vi "Logger Remove Last Log Element.vi"(8 "error in (no error)":errorcluster, 11 "LoggerRef In":T1) -> (0 "error out":errorcluster, 2 "Element Removed":string, 3 "LoggerRef Out":T1)   [LabVIEW 2014]
uses:
  LoggerRef.ctl
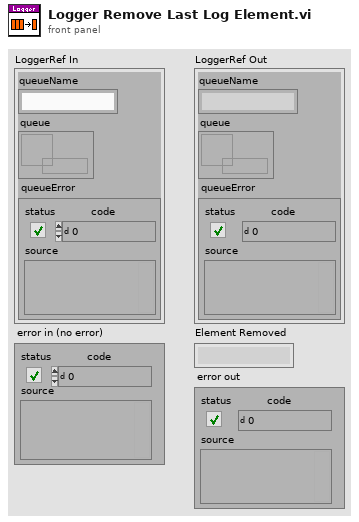
[diagram p1: front panel]
types:
  T1 = typedef "LoggerRef.ctl" = cluster{"queueName":string, "queue":refnum<queue>, "queueError":errorcluster}
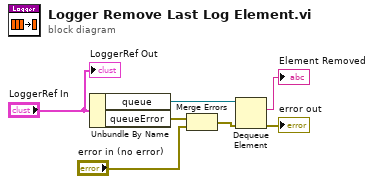
[diagram p0: block diagram]
diagram:
  n1 = Unbundle By Name("LoggerRef In") -> ("queue"=w4:refnum<queue>, "queueError"=w7:errorcluster)
  n2 = Merge Errors(w7, "error in (no error)") -> (w3:errorcluster)
  n3 = Dequeue Element(queue=w4, error in (no error)=w3) -> (element=→"Element Removed":string, error out=→"error out":errorcluster)  [unwired: 1 in, 2 out]
  "LoggerRef Out" <- "LoggerRef In"
